vi "Do-Fft.vi"(10 "FFT size":i32=-1, 11 "X":cdb[](array[numeric])) -> (3 "FFT {X}":cdb[](array[numeric]))   [LabVIEW 2014]
uses:
  <vilib>/Analysis/2dsp.llb/Complex FFT.vi
  <vilib>/Analysis/NI_AALPro.lvlib
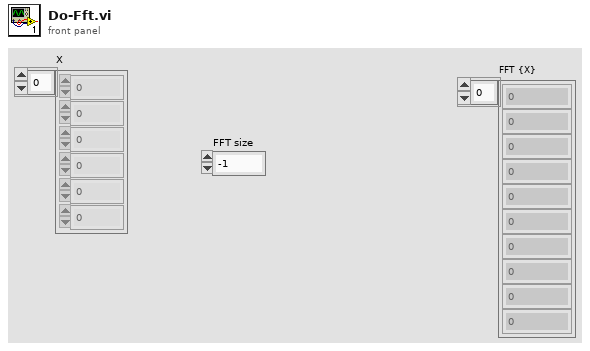
[diagram p1: front panel]
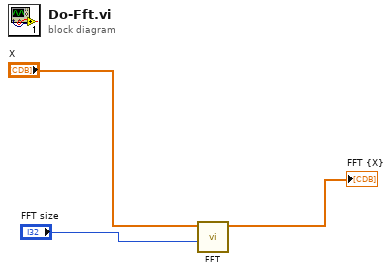
[diagram p0: block diagram]
diagram:
  n1 = call-poly <vilib>:"FFT.vi"("FFT size"="FFT size", "X"="X") -> ("FFT {X}"=→"FFT {X}":cdb[])  [unwired: 8 in, 1 out]
